vi "torque -- calc field div torque.vi"(4 "angle offset":dbl, 6 "parabola":T2, 7 "torque transformations":T1, 8 "angle":dbl, 10 "torque":dbl, 11 "field":dbl) -> (1 "transformed Y":dbl, 3 "field out":dbl)   [LabVIEW 2012]
uses:
  polynomial - bilinear.ctl
  torque transformation selector.ctl
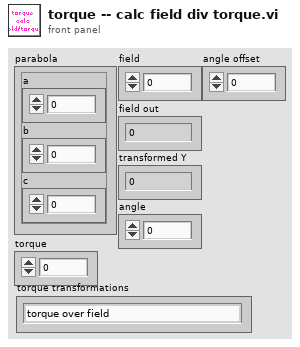
[diagram p1: front panel]
types:
  T1 = typedef "torque transformation selector.ctl" = enum16{"torque over field", "torque over field vs Hcos theta", "chi_torque vs Hcos theta"}
  T2 = typedef "polynomial - bilinear.ctl" = cluster{"a":dbl, "b":dbl, "c":dbl}
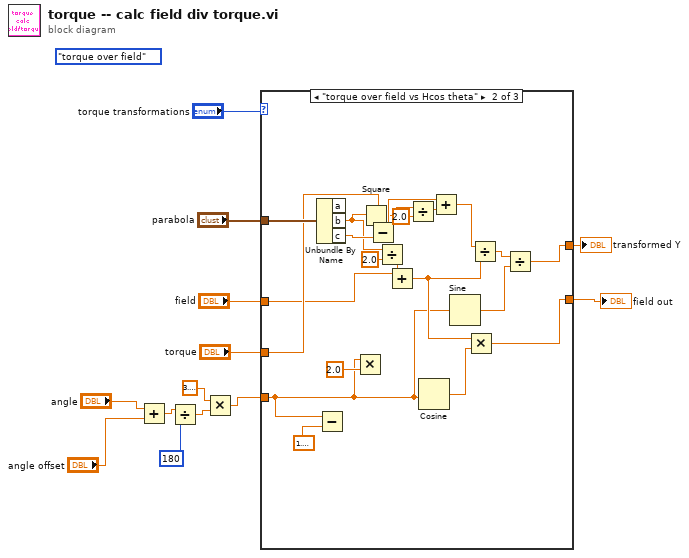
[diagram p0: block diagram]
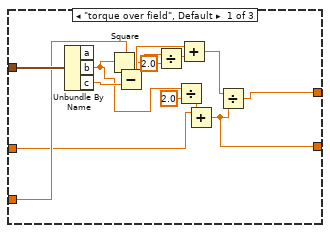
[diagram p2: hidden frame]
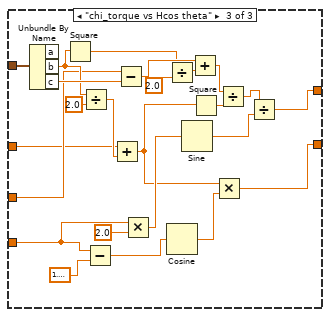
[diagram p3: hidden frame]
diagram:
  (unwired) torque_transformation_selector."torque over field" ("torque transformations")
  n1 = Add(x="angle", y="angle offset") -> (x+y=w1:dbl)
  n2 = Divide(x=w1, y=180) -> (x/y=w6:dbl)
  n3 = Multiply(x=3.141592653589793, y=w6) -> (x*y=w4:dbl)
  n4 = case shown="\"torque over field vs Hcos theta\"" "torque transformations" {
    tunnel: "parabola" -> [w18 w39 w63]
    tunnel: "field" -> [w15 w37 w61]
    tunnel: [w17 w29 w54] -> w11
    tunnel: "torque" -> [w16 w38 w62]
    tunnel: [w14 w35 w59] -> w8
    tunnel: w4 -> [_ w28 w53]
    frame "torque over field", Default {
      n5 = Unbundle By Name(w18) -> ("b"=w21:dbl, "c"=w27:dbl)  [unwired: 1 out]
      n6 = Square(x=w21) -> (x^2=w25:dbl)
      n7 = Subtract(x=w16, y=w27) -> (x-y=w26:dbl)
      n8 = Divide(x=w25, y=2.0) -> (x/y=w23:dbl)
      n9 = Divide(x=w21, y=2.0) -> (x/y=w20:dbl)
      n10 = Add(x=w26, y=w23) -> (x+y=w19:dbl)
      n11 = Add(x=w15, y=w20) -> (x+y=w14:dbl)
      n12 = Divide(x=w19, y=w14) -> (x/y=w17:dbl)
    }
    frame "torque over field vs Hcos theta" {
      n13 = Unbundle By Name(w39) -> ("b"=w42:dbl, "c"=w48:dbl)  [unwired: 1 out]
      n14 = Subtract(x=w28, y=1.5707963267948966) -> ()  [unwired: 1 out]
      n15 = Multiply(x=w28, y=2.0) -> ()  [unwired: 1 out]
      n16 = Square(x=w42) -> (x^2=w46:dbl)
      n17 = Subtract(x=w38, y=w48) -> (x-y=w47:dbl)
      n18 = Divide(x=w42, y=2.0) -> (x/y=w41:dbl)
      n19 = Add(x=w37, y=w41) -> (x+y=w33:dbl)
      n20 = Divide(x=w46, y=2.0) -> (x/y=w44:dbl)
      n21 = Cosine(x=w28) -> (cos(x)=w36:dbl)
      n22 = Add(x=w47, y=w44) -> (x+y=w40:dbl)
      n23 = Sine(x=w28) -> (sin(x)=w30:dbl)
      n24 = Multiply(x=w33, y=w36) -> (x*y=w35:dbl)
      n25 = Divide(x=w40, y=w33) -> (x/y=w31:dbl)
      n26 = Divide(x=w31, y=w30) -> (x/y=w29:dbl)
    }
    frame "chi_torque vs Hcos theta" {
      n27 = Unbundle By Name(w63) -> ("b"=w66:dbl, "c"=w72:dbl)  [unwired: 1 out]
      n28 = Square(x=w66) -> (x^2=w70:dbl)
      n29 = Divide(x=w66, y=2.0) -> (x/y=w65:dbl)
      n30 = Subtract(x=w53, y=1.5707963267948966) -> (x-y=w51:dbl)
      n31 = Add(x=w61, y=w65) -> (x+y=w49:dbl)
      n32 = Subtract(x=w62, y=w72) -> (x-y=w71:dbl)
      n33 = Multiply(x=w53, y=2.0) -> (x*y=w57:dbl)
      n34 = Divide(x=w70, y=2.0) -> (x/y=w68:dbl)
      n35 = Cosine(x=w51) -> (cos(x)=w60:dbl)
      n36 = Sine(x=w57) -> (sin(x)=w55:dbl)
      n37 = Add(x=w71, y=w68) -> (x+y=w64:dbl)
      n38 = Square(x=w49) -> (x^2=w50:dbl)
      n39 = Multiply(x=w49, y=w60) -> (x*y=w59:dbl)
      n40 = Divide(x=w64, y=w50) -> (x/y=w56:dbl)
      n41 = Divide(x=w56, y=w55) -> (x/y=w54:dbl)
    }
  }
  "field out" <- w8
  "transformed Y" <- w11
